vi "HistoricMaxMagnitude.vi"(1 "Reset":bool, 2 "Value":dbl) -> (0 "Max":dbl)   [LabVIEW 2017]
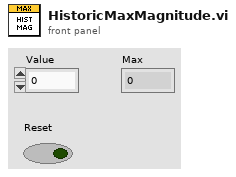
[diagram p1: front panel]
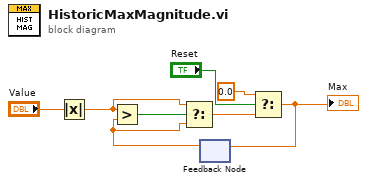
[diagram p0: block diagram]
diagram:
  n1 = Absolute Value(x="Value") -> (abs(x)=w7:dbl)
  n2 = feedback #1() -> (w6:dbl)  [unwired: 1 in]
  n3 = Greater?(x=w7, y=w6) -> (0:w8:bool)
  n4 = Select(t=w7, s=w8, f=w6) -> (s? t:f=w5:dbl)
  n5 = Select(t=0.0, s="Reset", f=w5) -> (s? t:f=w2:dbl)
  "Max" <- w2
  n6 = feedback-in #1(w2) -> ()
